vi "configureImageTriggering.vi"(8 "error in (no error)":errorcluster, 9 "Number of Images":dbl, 10 "Triggering":T1, 11 "CameraAcquisitor in":refnum<class "CameraAcquisitor.lvclass">) -> (0 "error out":errorcluster, 3 "CameraAcquisitor out":refnum<class "CameraAcquisitor.lvclass">)   [LabVIEW 2009, in "Hardware.lvlib" / "Channels.lvlib" / "CameraAcquisitor.lvclass"]
uses:
  CameraAcquisitor.lvclass
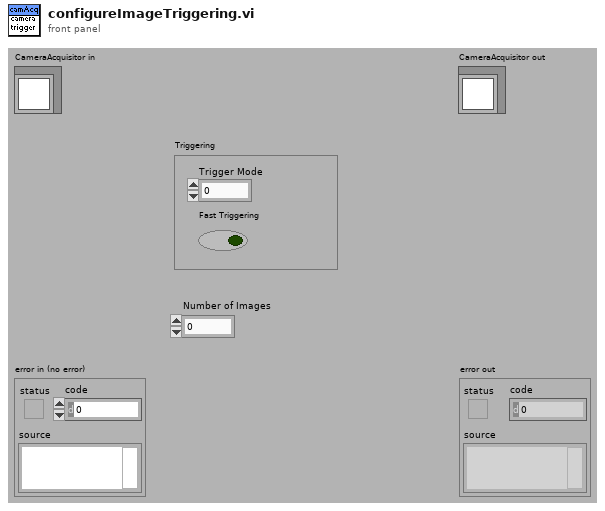
[diagram p1: front panel]
types:
  T1 = cluster{"Trigger Mode":dbl, "Fast Triggering":bool}
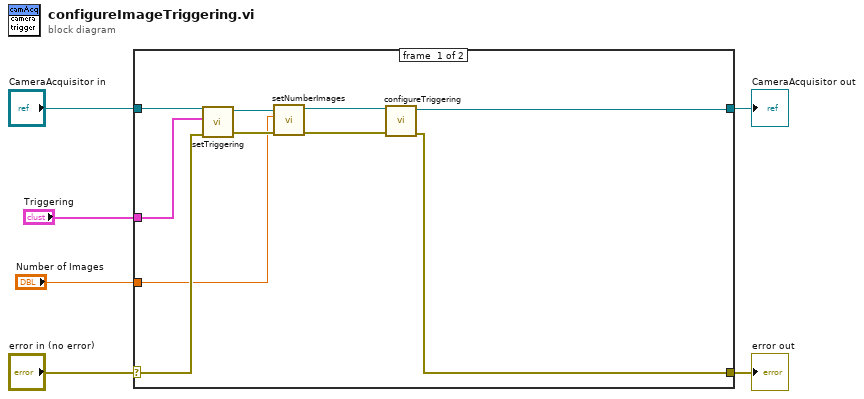
[diagram p0: block diagram]
diagram:
  n1 = case shown="No Error" "error in (no error)" {
    selector: "error in (no error)" -> [w14 w18]
    tunnel: [w12 w18] -> w5
    tunnel: [w13 w17] -> w3
    tunnel: "CameraAcquisitor in" -> [w16 w17]
    tunnel: "Triggering" -> [w15 _]
    tunnel: "Number of Images" -> [w9 _]
    frame #0 {
      n2 = call-dynamic "setTriggering.vi"("error in (no error)"=w14, "Triggering"=w15, "CameraAcquisitor.lvclass in"=w16) -> ("error out"=w10:errorcluster, "CameraAcquisitor.lvclass out"=w11:refnum<class "CameraAcquisitor.lvclass">)  [unwired: 7 in]
      n3 = call-dynamic "setNumberImages.vi"("error in (no error)"=w10, "Number of Images"=w9, "CameraAcquisitor.lvclass in"=w11) -> ("error out"=w8:errorcluster, "CameraAcquisitor.lvclass out"=w7:refnum<class "CameraAcquisitor.lvclass">)  [unwired: 7 in]
      n4 = call-dynamic "configureTriggering.vi"("error in (no error)"=w8, "CameraAcquisitor in"=w7) -> ("error out"=w12:errorcluster, "CameraAcquisitor out"=w13:refnum<class "CameraAcquisitor.lvclass">)  [unwired: 8 in]
    }
    frame #1 {
    }
  }
  "error out" <- w5
  "CameraAcquisitor out" <- w3
